vi "PopUp.vi"(8 "error in (no error)":errorcluster, 10 "String":string, 11 "My First Actor in":refnum<class "My First Actor.lvclass">) -> (0 "error out":errorcluster, 3 "My First Actor out":refnum<class "My First Actor.lvclass">)   [LabVIEW 2019, in "My First Actor.lvlib" / "My First Actor.lvclass"]
uses:
  My First Actor.lvclass
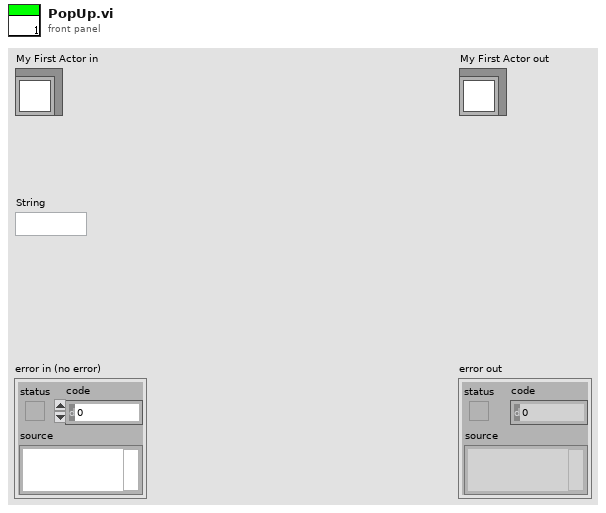
[diagram p1: front panel]
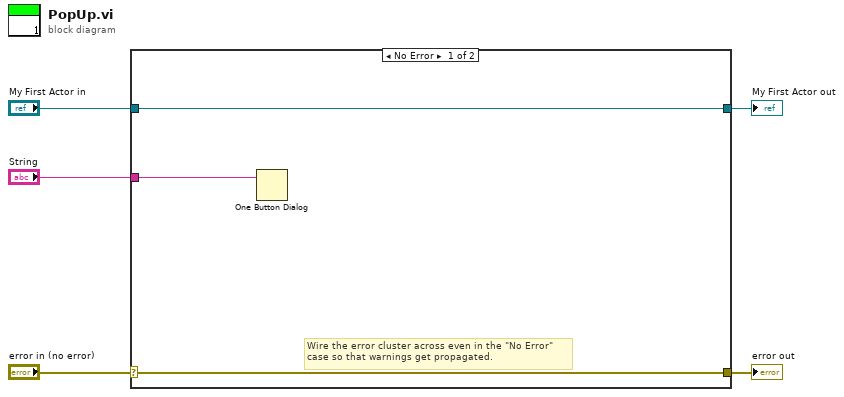
[diagram p0: block diagram]
diagram:
  n1 = case shown="No Error" "error in (no error)" {
    selector: "error in (no error)" -> [w7 w10]
    tunnel: [w7 w10] -> w4
    tunnel: [w8 w9] -> w2
    tunnel: "My First Actor in" -> [w8 w9]
    tunnel: "String" -> [w6 _]
    frame No Error {
      # "Wire the error cluster across even in the \"No Error\"\ncase so that warnings get propagated."
      n2 = One Button Dialog(message=w6) -> ()  [unwired: 1 in, 1 out]
    }
    frame Error {
    }
  }
  "error out" <- w4
  "My First Actor out" <- w2
